vi "Random Competition.vi"() -> ()   [LabVIEW 2019]
panel:
  out "Winner B":bool
  out "Tie":bool
  out "Winner A":bool
  out "Points B":i32
  out "Points A":i32
  out "Random Number B":dbl
  out "Random Number A":dbl
  in  "Number of Iterations":i32
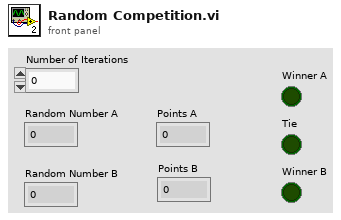
[diagram p1: front panel]
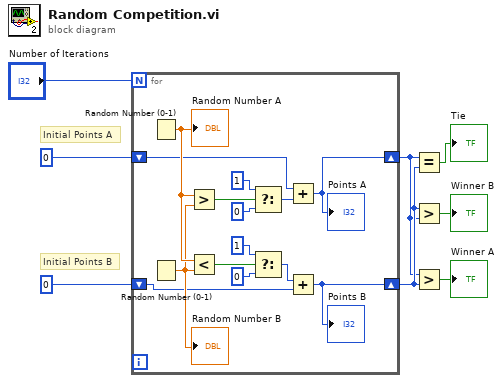
[diagram p0: block diagram]
diagram:
  # "Initial Points A"
  # "Initial Points B"
  n1 = for {
    N: "Number of Iterations" -> [_]
    shift-right: [w19] -> w2
    shift-left: 0 -> [w10]
    shift-right: [w11] -> w3
    shift-left: 0 -> [w9]
    n2 = Random Number (0-1)() -> (number: 0 to 1=w14:dbl)
    "Random Number A" <- w14
    n3 = Random Number (0-1)() -> (number: 0 to 1=w13:dbl)
    "Random Number B" <- w13
    n4 = Greater?(x=w14, y=w13) -> (0:w22:bool)
    n5 = Less?(x=w14, y=w13) -> (x < y?=w15:bool)
    n6 = Select(t=1, s=w22, f=0) -> (s? t:f=w20:i32)
    n7 = Select(t=1, s=w15, f=0) -> (s? t:f=w12:i32)
    n8 = Add(x=w10, y=w20) -> (x+y=w19:i32)
    "Points A" <- w19
    n9 = Add(x=w12, y=w9) -> (x+y=w11:i32)
    "Points B" <- w11
  }
  n10 = Equal?(x=w2, y=w3) -> (x = y?=→"Tie":bool)
  n11 = Greater?(x=w3, y=w2) -> (0:→"Winner B":bool)
  n12 = Greater?(x=w2, y=w3) -> (0:→"Winner A":bool)
